vi "Set Polymorphic.vi"   [LabVIEW 2020, in "NI_VIAnCFGDataStructure.lvlib" / "Tree.lvclass"]
doc: "Polymorphic instance of the Set method. Select the appropraite instance to work with or allow this method to adapt automatically."
uses:
  <vilib>/addons/analyzer/VIAnCFGDataStructure/Tree Manager/Tree.lvclass
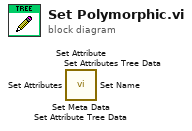
[diagram p0: block diagram]
diagram:
  n1 = call <vilib>:"Set Meta Data.vi"() -> ()  [unwired: 10 in, 2 out]
  n2 = call <vilib>:"Set Attributes Tree Data.vi"() -> ()  [unwired: 9 in, 3 out]
  n3 = call <vilib>:"Set Attributes.vi"() -> ()  [unwired: 9 in, 3 out]
  n4 = call <vilib>:"Set Name.vi"() -> ()  [unwired: 10 in, 2 out]
  n5 = call <vilib>:"Set Attribute Tree Data.vi"() -> ()  [unwired: 9 in, 3 out]
  n6 = call <vilib>:"Set Attribute.vi"() -> ()  [unwired: 9 in, 3 out]
